vi "Reorder 2D Data.vi"(8 "error in (no error)":errorcluster, 10 "Header Order[]":string[](array[string]) caption="Header Order[] (Optional)", 11 "SLL Table in":refnum<class "SLL Table.lvclass">) -> (0 "error out":errorcluster, 1 "2D Data Out[][]":string[][](array[string]), 2 "Headers Out[]":string[](array[string]), 3 "SLL Table out":refnum<class "SLL Table.lvclass">)   [LabVIEW 2014, in "SLL Table.lvclass"]
doc: "Get 2D Data in the column order you want. Headers is optional."
uses:
  SLL Table.lvclass
  SLL Table.lvclass/SLL Table.ctl
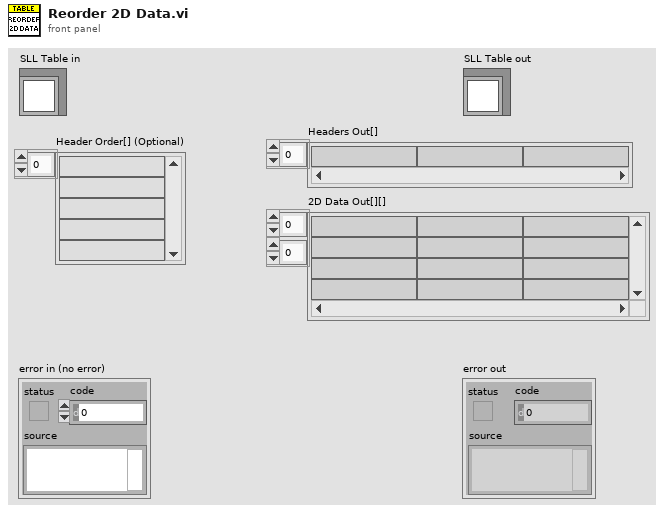
[diagram p1: front panel]
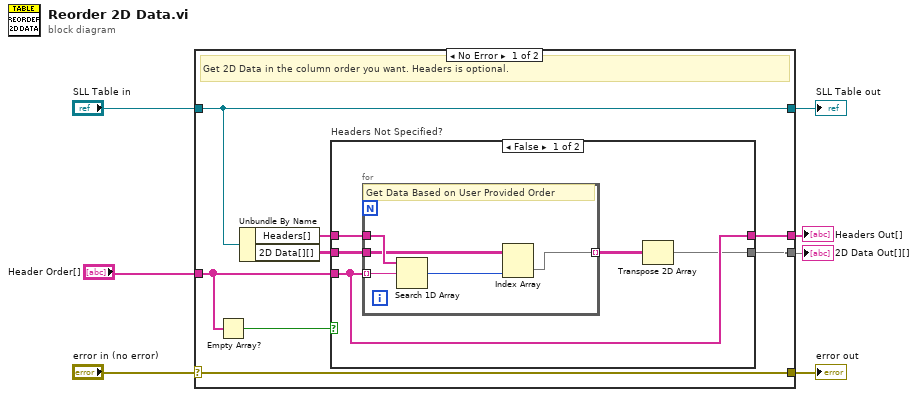
[diagram p0: block diagram]
diagram:
  n1 = case shown="No Error" "error in (no error)" {
    selector: "error in (no error)" -> [w15 w29]
    tunnel: [w15 w29] -> w6
    tunnel: [w14 w28] -> w4
    tunnel: "SLL Table in" -> [w14 w28]
    tunnel: [w10 _] -> w3
    tunnel: [w9 _] -> w2
    tunnel: "Header Order[]" -> [w8 _]
    frame No Error {
      # "Get 2D Data in the column order you want. Headers is optional."
      n2 = Empty Array?(array=w8) -> (empty?=w11:bool)
      n3 = Unbundle By Name(w14) -> ("Headers[]"=w13:string[], "2D Data[][]"=w12:string[][])
      n4 = case "Headers Not Specified?" shown="False" w11 {
        tunnel: w13 -> [w20 w27]
        tunnel: w12 -> [w19 w26]
        tunnel: [w17 w27] -> w10
        tunnel: [w16 w26] -> w9
        tunnel: w8 -> [w17 _]
        frame False {
          n5 = for {
            tunnel: w17 -> [w24] mode=indexing
            tunnel: w20 -> [w25]
            tunnel: w19 -> [w23]
            tunnel: [w21] -> w18 mode=indexing
            # "Get Data Based on User Provided Order"
            n6 = Search 1D Array(1D array=w25, element=w24) -> (index of element=w22:i32)  [unwired: 1 in]
            n7 = Index Array(array=w23, index (col)=w22) -> (element=w21:string[])  [unwired: 1 in]
          }
          n8 = Transpose 2D Array(2D array=w18) -> (transposed array=w16:string[][])
        }
        frame True {
        }
      }
    }
    frame Error {
    }
  }
  "error out" <- w6
  "SLL Table out" <- w4
  "Headers Out[]" <- w3
  "2D Data Out[][]" <- w2
